vi "calcEncoderPosition.vi"(8 "error in (no error)":errorcluster, 11 "Encoder in":refnum<class "Encoder.lvclass">) -> (0 "error out":errorcluster, 3 "Encoder out":refnum<class "Encoder.lvclass">)   [LabVIEW 2013, in "Encoder.lvclass"]
uses:
  Encoder.lvclass
  Encoder.lvclass/Encoder.ctl
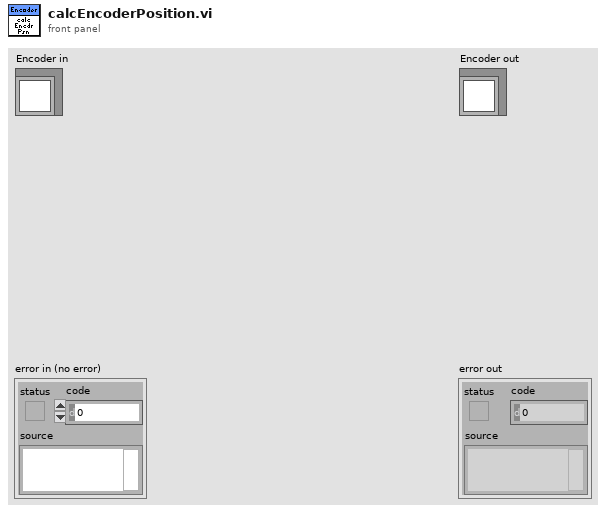
[diagram p1: front panel]
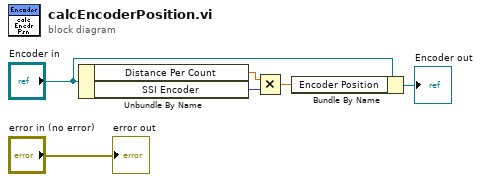
[diagram p0: block diagram]
diagram:
  n1 = Unbundle By Name("Encoder in") -> ("Distance Per Count"=w5:dbl[unit], "SSI Encoder"=w4:i32)
  n2 = Multiply(x=w5, y=w4) -> (x*y=w1:dbl[unit])
  n3 = Bundle By Name(cluster="Encoder in", "Encoder Position"=w1) -> (→"Encoder out":refnum<class "Encoder.lvclass">)
  "error out" <- "error in (no error)"
